vi "AUTO_Queue_States.vi"(7 "QUEUE ST":T2=enum."CLOSE Q", 8 "error in":errorcluster, 11 "AUTO ST IN":T1[](array[typedef])=[enum."Int"]) -> (0 "error OUT":errorcluster, 3 "AUTO ST":T1)   [LabVIEW 2017]
uses:
  Controls/QUEUE_STATES.ctl
  Controls/AUTO_St.ctl
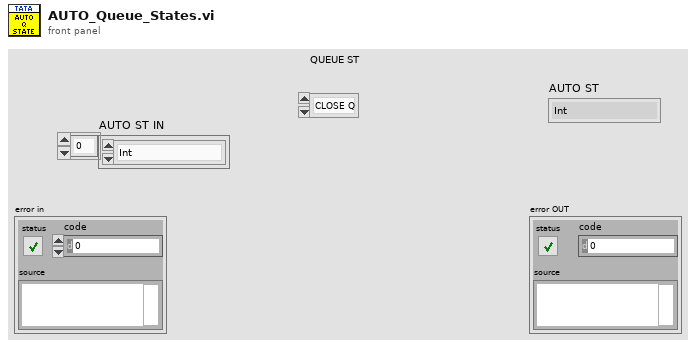
[diagram p1: front panel]
types:
  T1 = typedef "AUTO_St.ctl" = enum16{"Int", "Int2", "CLUSTER_UPDATE", "WAIT", "AUTO_CYCLE_RUNNING_ST1", "SCAN_STATION_1", "STATION_1_CMPLT_OK", "STATION_1_ABORT_NG", "SCAN_STATION_2", "LOAD CELL PICK UP", "AUTO_CYCLE_COMP_ST2", "AUTO_CYCLE_ABORT_ST2", "PRINT", "CYCLE_DISTANCE FAIL_ST2", "AUTO_CYC_START_ST2", "Error_Handler", "Stop"}
  T2 = typedef "QUEUE_STATES.ctl" = enum16{"CREATE Q", "EN Q", "DE Q", "CLOSE Q"}
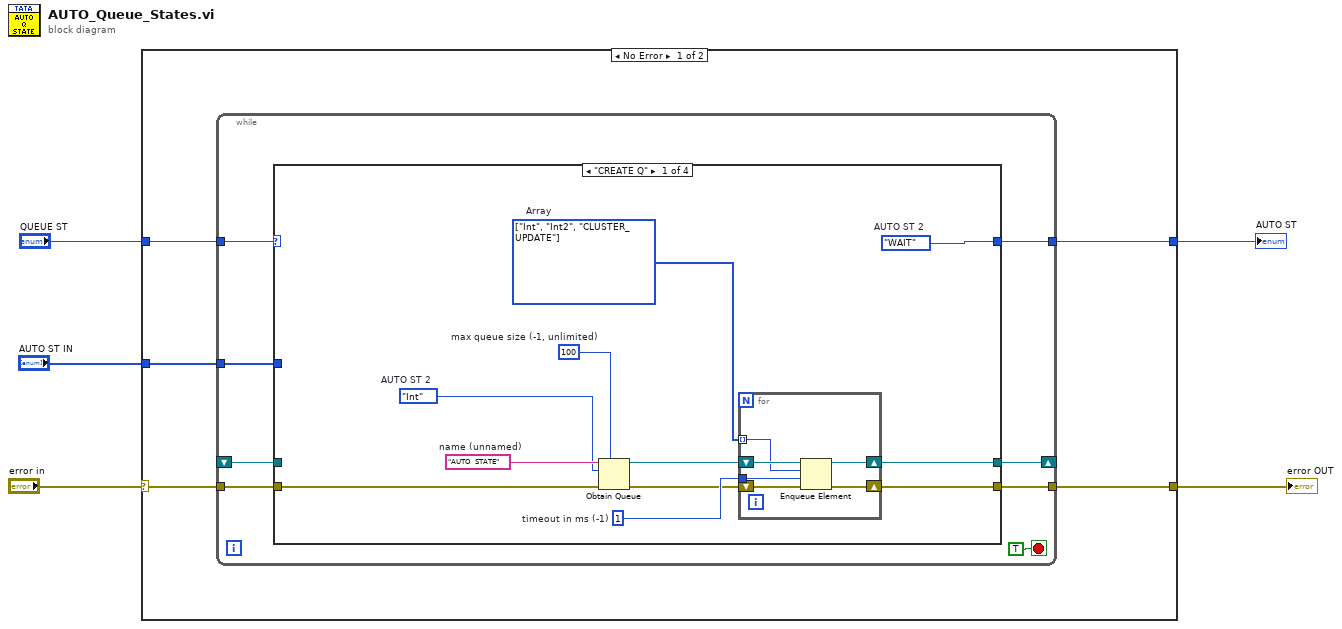
[diagram p0: block diagram]
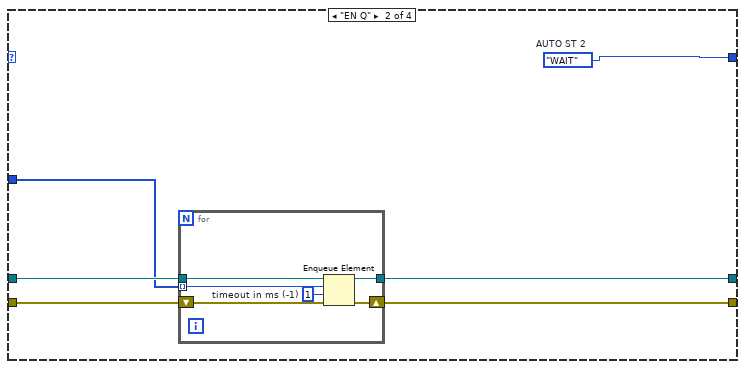
[diagram p2: hidden frame]
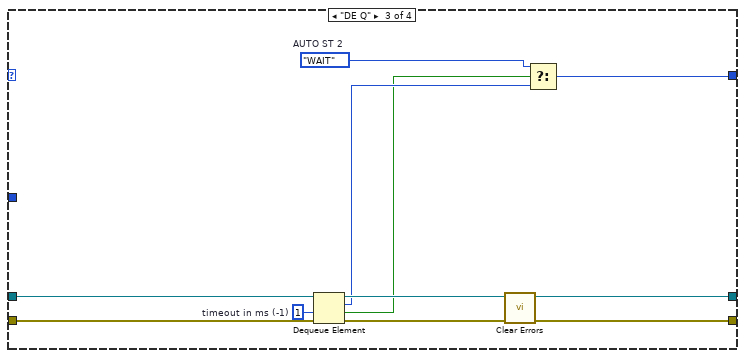
[diagram p3: hidden frame]
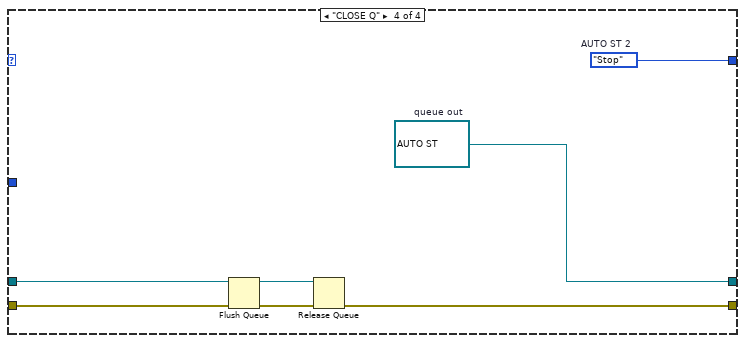
[diagram p4: hidden frame]
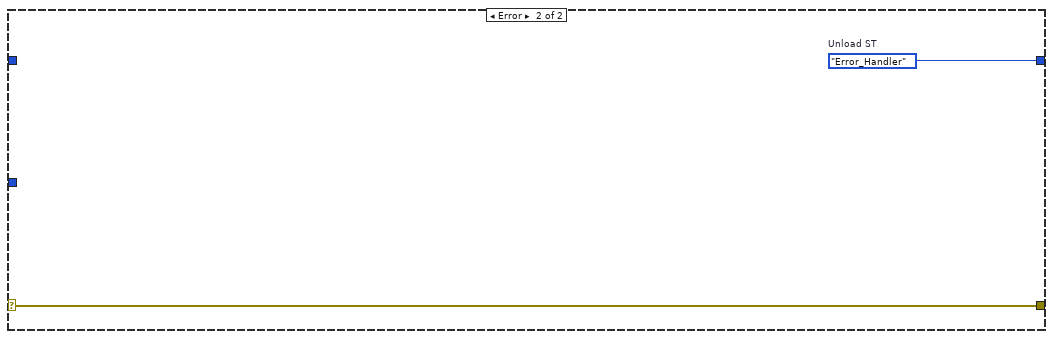
[diagram p5: hidden frame]
diagram:
  n1 = case shown="No Error" "error in" {
    selector: "error in" -> [w10 w66]
    tunnel: [w9 w66] -> w4
    tunnel: [w8 w65] -> w1
    tunnel: "QUEUE ST" -> [w7 _]
    tunnel: "AUTO ST IN" -> [w6 _]
    frame No Error {
      n2 = while {
        tunnel: w10 -> [w18]
        tunnel: [w16] -> w9
        tunnel: [w11] -> w8
        tunnel: w7 -> [w15]
        shift-right: [w14] -> _
        shift-left: _ -> [w13]
        tunnel: w6 -> [w12]
        stop <- TRUE stop-if-true
        n3 = case shown="\"CREATE Q\"" w15 {
          tunnel: w18 -> [w29 w41 w57 w63]
          tunnel: [w22 w40 w49 w64] -> w16
          tunnel: [w24 w38 w54 w58] -> w14
          tunnel: w13 -> [_ w39 w55 w61]
          tunnel: w12 -> [_ w37 _ _]
          tunnel: [w21 w36 w51 w59] -> w11
          frame "CREATE Q" {
            w19 = T1[] [enum."Int", enum."Int2", enum."CLUSTER_UPDATE"] items=["Int", "Int2", "CLUSTER_UPDATE", "WAIT", "AUTO_CYCLE_RUNNING_ST1", "SCAN_STATION_1", "STATION_1_CMPLT_OK", "STATION_1_ABORT_NG", "SCAN_STATION_2", "LOAD CELL PICK UP", "AUTO_CYCLE_COMP_ST2", "AUTO_CYCLE_ABORT_ST2", "PRINT", "CYCLE_DISTANCE FAIL_ST2", "AUTO_CYC_START_ST2", "Error_Handler", "Stop"]  # Array
            w20 = AUTO_St."Int"  # AUTO ST 2
            w21 = AUTO_St."WAIT"  # AUTO ST 2
            w26 = 1  # timeout in ms (-1)
            w27 = 100  # max queue size (-1, unlimited)
            w28 = "AUTO  STATE"  # name (unnamed)
            n4 = Obtain Queue(max queue size (-1, unlimited)=w27, name (unnamed)=w28, element data type=w20, error in (no error)=w29) -> (queue out=w25:refnum<queue>, error out=w23:errorcluster)  [unwired: 1 in, 1 out]
            n5 = for {
              tunnel: w26 -> [w35]
              tunnel: w19 -> [w30] mode=indexing
              shift-right: [w33] -> w24
              shift-left: w25 -> [w34]
              shift-right: [w31] -> w22
              shift-left: w23 -> [w32]
              n6 = Enqueue Element(queue=w34, element=w30, timeout in ms (-1)=w35, error in (no error)=w32) -> (queue out=w33:refnum<queue>, error out=w31:errorcluster)  [unwired: 1 out]
            }
          }
          frame "EN Q" {
            w36 = AUTO_St."WAIT"  # AUTO ST 2
            n7 = for {
              tunnel: w39 -> [w45]
              tunnel: [w44] -> w38
              tunnel: w37 -> [w43] mode=indexing
              shift-right: [w46] -> w40
              shift-left: w41 -> [w47]
              w42 = 1  # timeout in ms (-1)
              n8 = Enqueue Element(queue=w45, element=w43, timeout in ms (-1)=w42, error in (no error)=w47) -> (queue out=w44:refnum<queue>, error out=w46:errorcluster)  [unwired: 1 out]
            }
          }
          frame "DE Q" {
            w48 = AUTO_St."WAIT"  # AUTO ST 2
            w53 = 1  # timeout in ms (-1)
            n9 = Dequeue Element(queue=w55, timeout in ms (-1)=w53, error in (no error)=w57) -> (queue out=w54:refnum<queue>, element=w52:T1, timed out?=w50:bool, error out=w56:errorcluster)
            n10 = call <vilib>:"Clear Errors.vi"("error in (no error)"=w56) -> ("error out"=w49:errorcluster)  [unwired: 5 in, 1 out]
            n11 = Select(t=w48, s=w50, f=w52) -> (s? t:f=w51:T1)
          }
          frame "CLOSE Q" {
            w58 = refnum<queue> refnum items=["Int", "Int2", "CLUSTER_UPDATE", "WAIT", "AUTO_CYCLE_RUNNING_ST1", "SCAN_STATION_1", "STATION_1_CMPLT_OK", "STATION_1_ABORT_NG", "SCAN_STATION_2", "LOAD CELL PICK UP", "AUTO_CYCLE_COMP_ST2", "AUTO_CYCLE_ABORT_ST2", "PRINT", "CYCLE_DISTANCE FAIL_ST2", "AUTO_CYC_START_ST2", "Error_Handler", "Stop"]  # queue out
            w59 = AUTO_St."Stop"  # AUTO ST 2
            n12 = Flush Queue(queue=w61, error in (no error)=w63) -> (queue out=w60:refnum<queue>, error out=w62:errorcluster)  [unwired: 1 out]
            n13 = Release Queue(queue=w60, error in (no error)=w62) -> (error out=w64:errorcluster)  [unwired: 1 in, 2 out]
          }
        }
      }
    }
    frame Error {
      w65 = AUTO_St."Error_Handler"  # Unload ST
    }
  }
  "error OUT" <- w4
  "AUTO ST" <- w1
